vi "Sender UI.vi"(8 "Error In":errorcluster, 9 "Transmission Type":T1, 10 "Transmission Data":string(combo)) -> (0 "Error Out":errorcluster)   [LabVIEW 2023, in "Sender.lvclass"]
uses:
  Sender.lvclass
  Controls/Message Type.ctl
  Controls/Queue Operation.ctl
  Controls/User Event Operations.ctl
  Controls/Messenger Data.ctl
  Controls/Type Class Ref.ctl
  Controls/Class DVR Ref.ctl
  Data/Data.lvclass
  Sender.lvclass/Sender.ctl
  Communication/Communication.lvclass
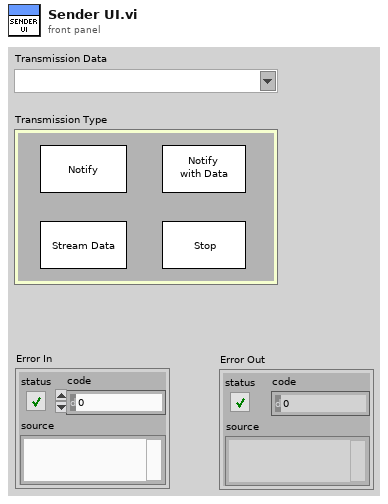
[diagram p1: front panel]
types:
  T1 = typedef "Message Type.ctl" = cluster{"Notify Only":bool, "Notify With Data":bool, "Stream Data":bool, "Hang Up":bool}
  T2 = typedef "Messenger Data.ctl" = cluster{"Message Data path":path, "Start Time":dbl, "Elapsed TIme":dbl, "Message Type":refnum<class "Communication.lvclass">, "Selected Message Data":string, "Selected Message Type":string, "Type DVR Ref":T3[], "Data DVR Ref":T4[], "Type DVR":refnum<data-value>, "Data DVR":refnum<data-value>, "Stream?":bool, "Wait Time":dbl, "Port Number":i32}
  T3 = typedef "Type Class Ref.ctl" = cluster{"Class Name":string, "Class DVR Ref":refnum<data-value>}
  T4 = typedef "Class DVR Ref.ctl" = cluster{"Class DVR Ref":refnum<data-value>, "Class Name":string}
  T5 = typedef "User Event Operations.ctl" = enum16{"Obtain", "Generate", "Destroy"}
  T6 = typedef "Queue Operation.ctl" = enum16{"Create & Enqueue N", "Enqueue N", "Dequeue", "Enstack N", "Flush", "Release"}
  T7 = enum8{"Enabled", "Disabled", "Disabled and Grayed Out"}
  T8 = typedef "Queue Element.ctl" = cluster{"State":string, "Data":variant}
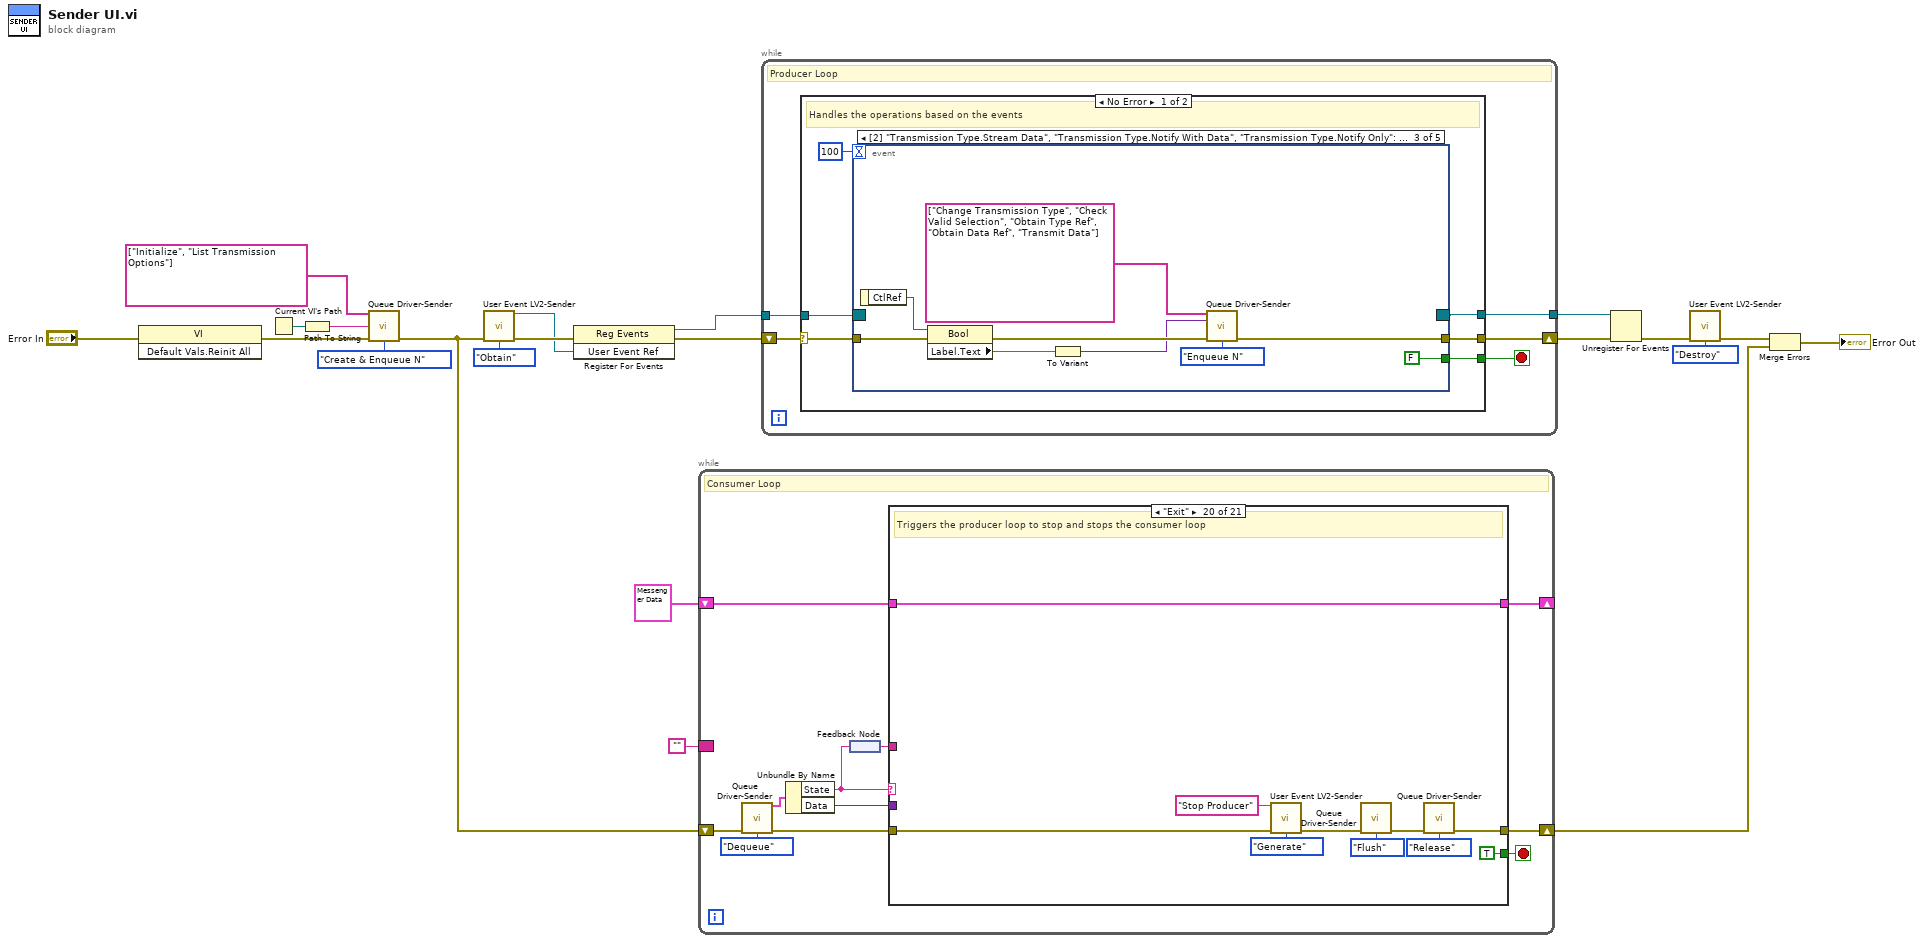
[diagram p0: block diagram]
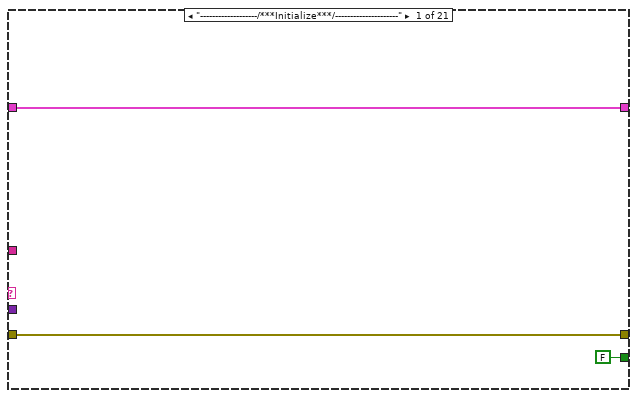
[diagram p2: hidden frame]
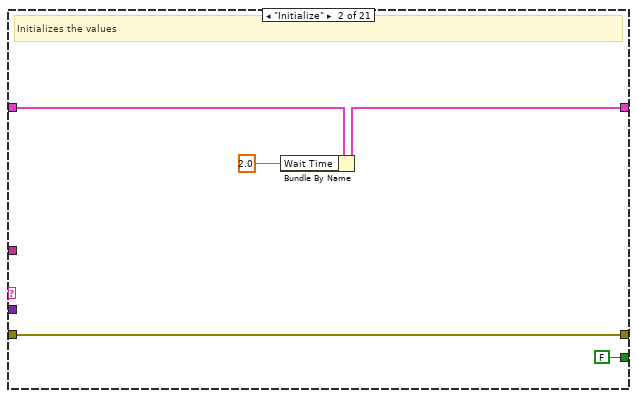
[diagram p3: hidden frame]
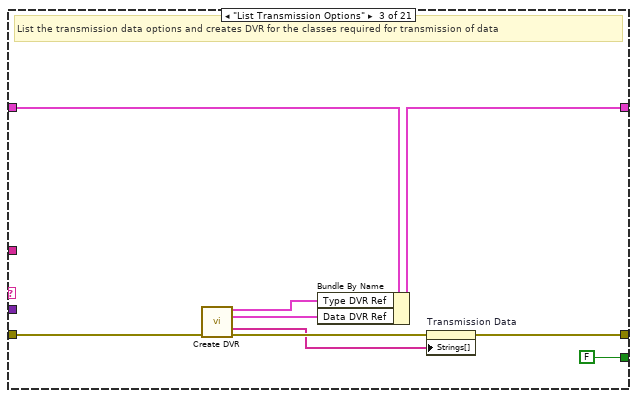
[diagram p4: hidden frame]
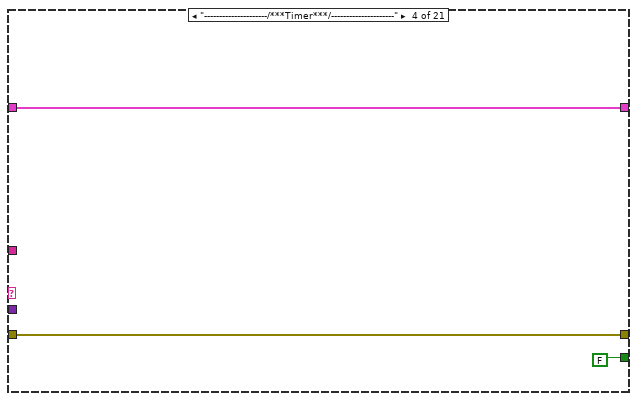
[diagram p5: hidden frame]
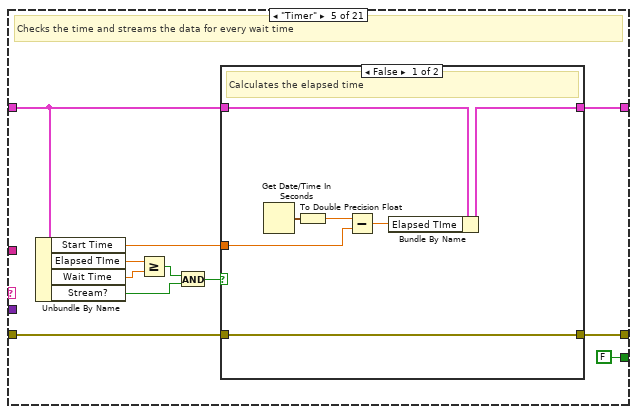
[diagram p6: hidden frame]
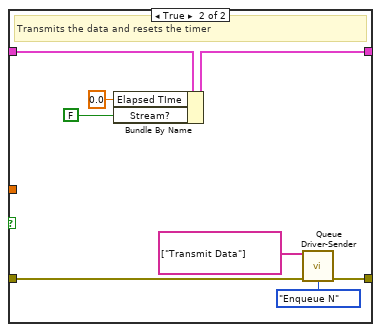
[diagram p7: hidden frame]
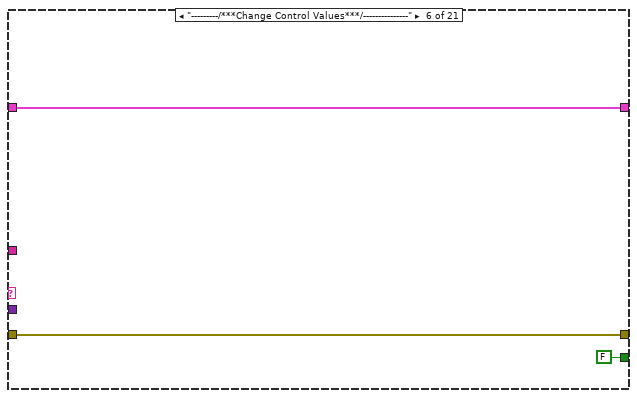
[diagram p8: hidden frame]
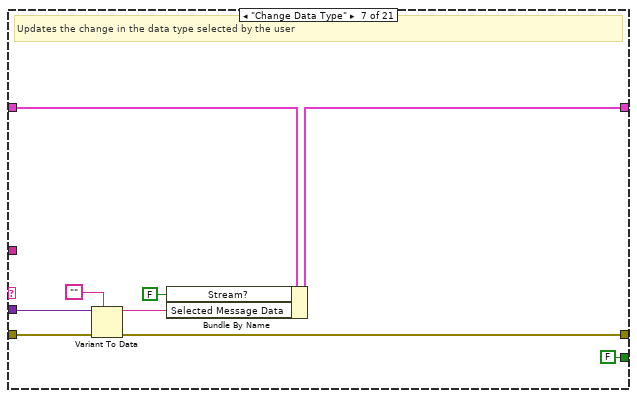
[diagram p9: hidden frame]
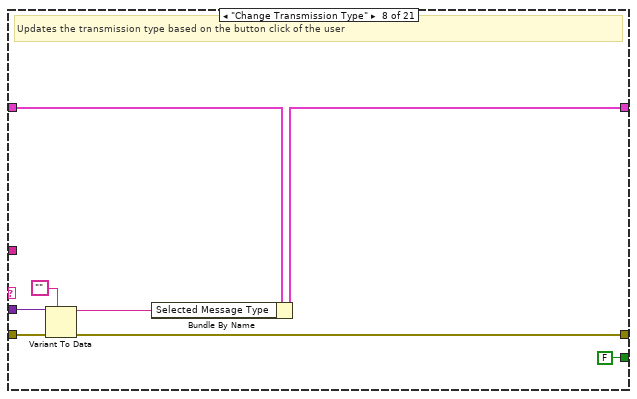
[diagram p10: hidden frame]
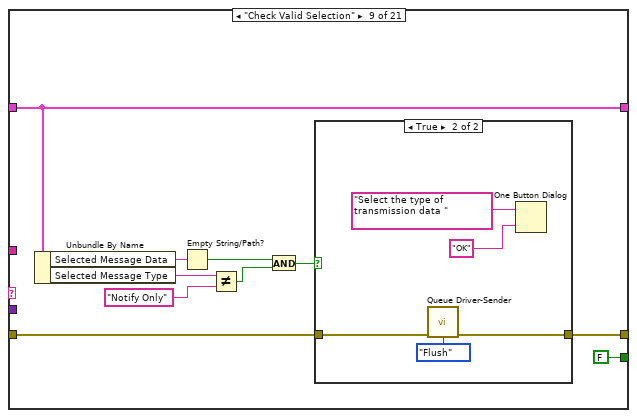
[diagram p11: hidden frame]
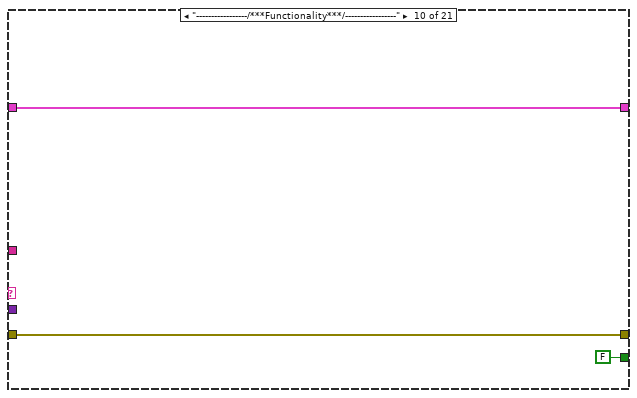
[diagram p13: hidden frame]
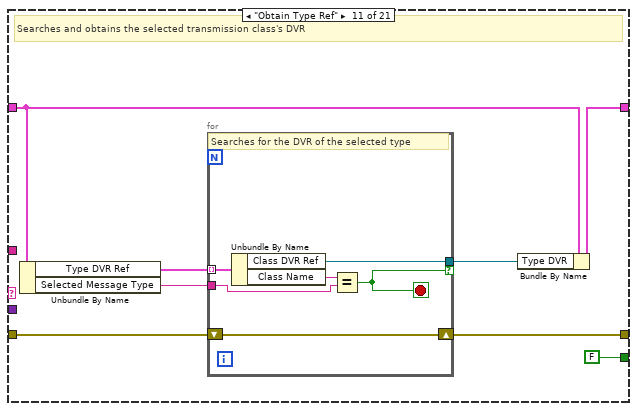
[diagram p14: hidden frame]
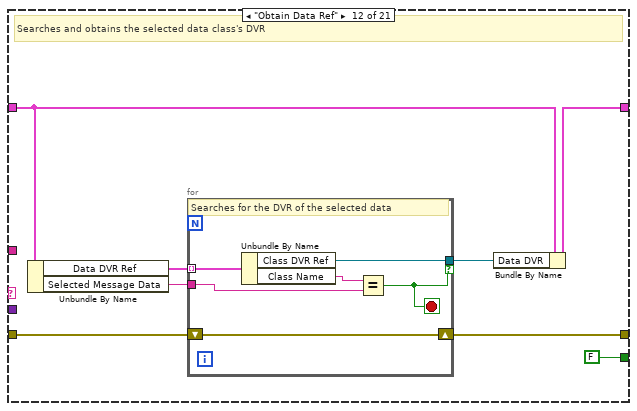
[diagram p15: hidden frame]
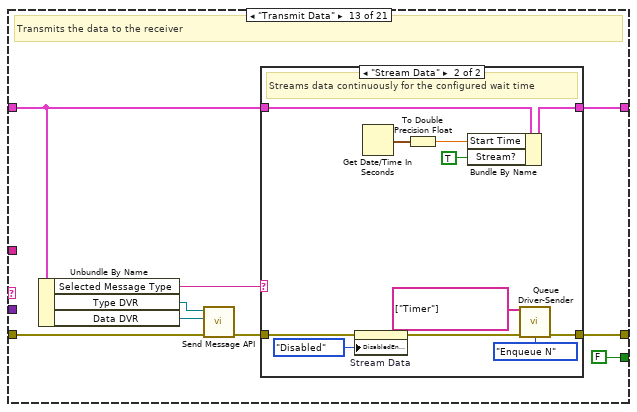
[diagram p16: hidden frame]
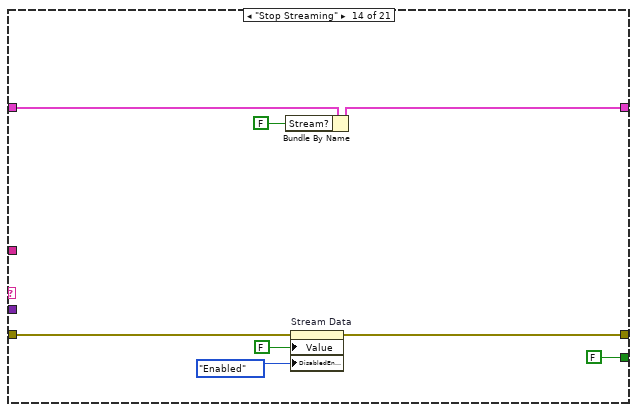
[diagram p18: hidden frame]
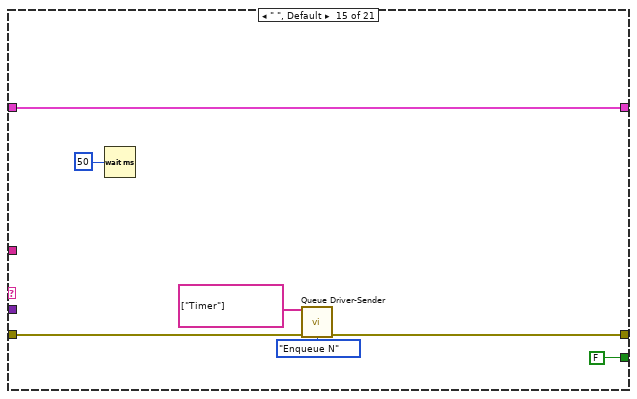
[diagram p19: hidden frame]
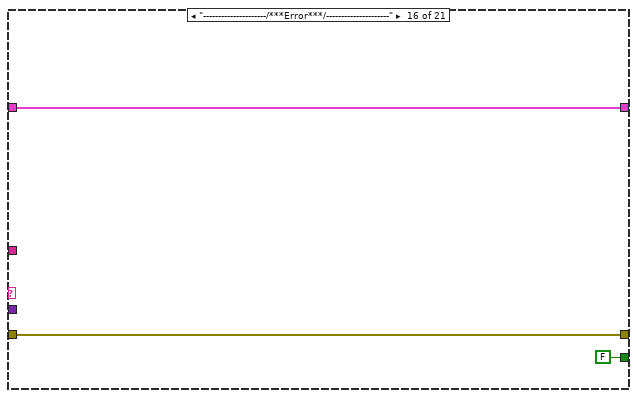
[diagram p20: hidden frame]
diagram:
  n1 = invoke class="VI" method="Default Vals.Reinit All"(error in="Error In") -> (error out=w1:errorcluster)  [unwired: 2 in, 2 out]
  n2 = Current VI's Path() -> (path=w3:path)
  n3 = Path To String(path=w3) -> (string=w2:string)
  n4 = call "Queue Driver-Sender.vi"("States[]"=string[] ["Initialize", "List Transmission Options"], "Queue Name"=w2, "Error In"=w1, "Queue Operation"=Queue_Operation."Create & Enqueue N") -> ("Error Out"=w13:errorcluster)  [unwired: 10 in, 1 out]
  n5 = call "User Event LV2-Sender.vi"("Error In"=w13, "Operation"=User_Event_Operations."Obtain") -> ("User Event Ref"=w11:refnum<user-event>, "Error Out"=w15:errorcluster)  [unwired: 12 in]
  n6 = register-events(error in=w15, w11) -> (reference out=w10:refnum<event-registration>, error out=w12:errorcluster)  [unwired: 1 in]
  n7 = while {
    shift-right: [w31] -> w16
    shift-left: w13 -> [w32]
    border: "" -> [_]
    shift-right: [w22] -> _
    shift-left: T2 {"Message Data path"=path "", "Start Time"=0.0, "Elapsed TIme"=0.0, "Message Type"=refnum, "Selected Message Data"="", "Selected Message Type"="", "Type DVR Ref"=[], "Data DVR Ref"=[], "Type DVR"=refnum, "Data DVR"=refnum, "Stream?"=FALSE, "Wait Time"=0.0, "Port Number"=0} -> [w23]
    stop <- w27 stop-if-true
    # "Consumer Loop"
    n8 = call "Queue Driver-Sender.vi"("Error In"=w32, "Queue Operation"=Queue_Operation."Dequeue") -> ("Dequeue Element"=w28:T8, "Error Out"=w30:errorcluster)  [unwired: 12 in]
    n9 = Unbundle By Name(w28) -> ("State"=w26:string, "Data"=w24:variant)
    n10 = feedback-in #1(w26) -> ()
    n11 = feedback #1() -> (w25:string)
    n12 = case shown="\"Exit\"" w26 {
      tunnel: w30 -> [w35 w39 w49 w52 w63 w81 w90 w98 w108 w117 w125 w139 w154 w175 w182 w185 w191 w220 w228 w238 w247]
      tunnel: [w35 w39 w41 w52 w62 w81 w84 w96 w105 w117 w124 w138 w150 w170 w179 w185 w188 w207 w228 w234 w245] -> w31
      tunnel: [FALSE FALSE FALSE FALSE FALSE FALSE FALSE FALSE FALSE FALSE FALSE FALSE FALSE FALSE FALSE FALSE FALSE FALSE FALSE TRUE FALSE] -> w27
      tunnel: w25 -> [_ _ _ _ _ _ _ _ _ _ _ _ _ _ _ _ w189 _ _ _ _]
      tunnel: w24 -> [_ _ _ _ _ _ w85 w95 _ _ _ _ _ _ _ _ _ w212 _ _ _]
      tunnel: w23 -> [w33 w38 w47 w51 w60 w80 w87 w97 w106 w115 w123 w137 w149 w174 w180 w183 w186 w219 w226 w229 w246]
      tunnel: [w33 w37 w45 w51 w59 w80 w86 w93 w106 w115 w119 w133 w151 w173 w180 w183 w186 w219 w226 w229 w246] -> w22
      frame "-------------------/***Initialize***/---------------------" {
      }
      frame "Initialize" {
        # "Initializes the values"
        n13 = Bundle By Name(cluster=w38, "Wait Time"=2.0) -> (w37:T2)
      }
      frame "List Transmission Options" {
        # "List the transmission data options and creates DVR for the classes required for transmission of data"
        n14 = call "Create DVR.vi"("Error In"=w49) -> ("Communication DVR Refs"=w44:T3[], "Data Type DVR Refs"=w43:T4[], "Data Types"=w42:string[], "Error Out"=w46:errorcluster)  [unwired: 10 in, 1 out]
        n15 = Bundle By Name(cluster=w47, "Type DVR Ref"=w44, "Data DVR Ref"=w43) -> (w45:T2)
        n16 = property on="Transmission Data" class="CmbBox"(error in=w46, "Strings[]"=w42) -> (error out=w41:errorcluster)  [unwired: 1 in, 1 out]
      }
      frame "---------------------/***Timer***/---------------------" {
      }
      frame "Timer" {
        # "Checks the time and streams the data for every wait time"
        n17 = Unbundle By Name(w60) -> ("Start Time"=w61:dbl, "Elapsed TIme"=w57:dbl, "Wait Time"=w53:dbl, "Stream?"=w54:bool)
        n18 = Greater Or Equal?(x=w57, y=w53) -> (x >= y?=w56:bool)
        n19 = And(x=w56, y=w54) -> (x .and. y?=w55:bool)
        n20 = case shown="False" w55 {
          tunnel: w63 -> [w69 w71]
          tunnel: [w69 w77] -> w62
          tunnel: w61 -> [w64 _]
          tunnel: [w68 w74] -> w59
          tunnel: w60 -> [w70 w78]
          frame False {
            # "Calculates the elapsed time"
            n21 = Get Date/Time In Seconds() -> (seconds since 1Jan1904=w67:timestamp)
            n22 = To Double Precision Float(number=w67) -> (double precision float=w65:dbl)
            n23 = Subtract(x=w65, y=w64) -> (x-y=w66:dbl)
            n24 = Bundle By Name(cluster=w70, "Elapsed TIme"=w66) -> (w68:T2)
          }
          frame True {
            # "Transmits the data and resets the timer"
            n25 = Bundle By Name(cluster=w78, "Elapsed TIme"=0.0, "Stream?"=FALSE) -> (w74:T2)
            n26 = call "Queue Driver-Sender.vi"("States[]"=string[] ["Transmit Data"], "Error In"=w71, "Queue Operation"=Queue_Operation."Enqueue N") -> ("Error Out"=w77:errorcluster)  [unwired: 11 in, 1 out]
          }
        }
      }
      frame "---------/***Change Control Values***/---------------" {
      }
      frame "Change Data Type" {
        # "Updates the change in the data type selected by the user"
        n27 = Variant To Data(error in=w90, type="", Variant=w85) -> (data=w83:string, error out=w84:errorcluster)
        n28 = Bundle By Name(cluster=w87, "Stream?"=FALSE, "Selected Message Data"=w83) -> (w86:T2)
      }
      frame "Change Transmission Type" {
        # "Updates the transmission type based on the button click of the user"
        n29 = Variant To Data(error in=w98, type="", Variant=w95) -> (data=w92:string, error out=w96:errorcluster)
        n30 = Bundle By Name(cluster=w97, "Selected Message Type"=w92) -> (w93:T2)
      }
      frame "Check Valid Selection" {
        n31 = Unbundle By Name(w106) -> ("Selected Message Data"=w104:string, "Selected Message Type"=w102:string)
        n32 = Empty String/Path?(string/path=w104) -> (empty?=w101:bool)
        n33 = Not Equal?(x=w102, y="Notify Only") -> (x != y?=w100:bool)
        n34 = And(x=w101, y=w100) -> (x .and. y?=w99:bool)
        n35 = case shown="True" w99 {
          tunnel: w108 -> [w109 w114]
          tunnel: [w109 w111] -> w105
          frame False {
          }
          frame True {
            n36 = call "Queue Driver-Sender.vi"("Error In"=w114, "Queue Operation"=Queue_Operation."Flush") -> ("Error Out"=w111:errorcluster)  [unwired: 12 in, 1 out]
            n37 = One Button Dialog(message="Select the type of transmission data ", button name ("OK")="OK") -> ()  [unwired: 1 out]
          }
        }
      }
      frame "-----------------/***Functionality***/-----------------" {
      }
      frame "Obtain Type Ref" {
        # "Searches and obtains the selected transmission class's DVR"
        n38 = Unbundle By Name(w123) -> ("Type DVR Ref"=w122:T3[], "Selected Message Type"=w121:string)
        n39 = for {
          shift-right: [w131] -> w124
          shift-left: w125 -> [w131]
          tunnel: w122 -> [w130] mode=indexing
          tunnel: w121 -> [w128]
          tunnel: [w127] -> w118 if=w126
          stop <- w126 stop-if-true
          # "Searches for the DVR of the selected type"
          n40 = Unbundle By Name(w130) -> ("Class DVR Ref"=w127:refnum<data-value>, "Class Name"=w129:string)
          n41 = Equal?(x=w129, y=w128) -> (x = y?=w126:bool)
        }
        n42 = Bundle By Name(cluster=w123, "Type DVR"=w118) -> (w119:T2)
      }
      frame "Obtain Data Ref" {
        # "Searches and obtains the selected data class's DVR"
        n43 = Unbundle By Name(w137) -> ("Data DVR Ref"=w136:T4[], "Selected Message Data"=w135:string)
        n44 = for {
          shift-right: [w145] -> w138
          shift-left: w139 -> [w145]
          tunnel: w136 -> [w144] mode=indexing
          tunnel: w135 -> [w141]
          tunnel: [w143] -> w132 if=w140
          stop <- w140 stop-if-true
          # "Searches for the DVR of the selected data"
          n45 = Unbundle By Name(w144) -> ("Class DVR Ref"=w143:refnum<data-value>, "Class Name"=w142:string)
          n46 = Equal?(x=w142, y=w141) -> (x = y?=w140:bool)
        }
        n47 = Bundle By Name(cluster=w137, "Data DVR"=w132) -> (w133:T2)
      }
      frame "Transmit Data" {
        # "Transmits the data to the receiver"
        n48 = Unbundle By Name(w149) -> ("Selected Message Type"=w148:string, "Type DVR"=w147:refnum<data-value>, "Data DVR"=w146:refnum<data-value>)
        n49 = call "Send Message API.vi"("error in (no error)"=w154, "Data DVR"=w146, "Type DVR"=w147) -> ("error out"=w152:errorcluster)  [unwired: 8 in]
        n50 = case shown="\"Stream Data\"" w148 {
          tunnel: w152 -> [w155 w167]
          tunnel: [w156 w166] -> w151
          tunnel: [w155 w163] -> w150
          tunnel: w149 -> [w156 w160]
          frame Default {
          }
          frame "Stream Data" {
            # "Streams data continuously for the configured wait time"
            n51 = property on="Stream Data" class="Bool (strict)"(error in=w167, "DisabledEnum"=T7."Disabled" ("Disabled")) -> (error out=w158:errorcluster)  [unwired: 1 in, 1 out]
            n52 = Get Date/Time In Seconds() -> (seconds since 1Jan1904=w164:timestamp)
            n53 = To Double Precision Float(number=w164) -> (double precision float=w165:dbl)
            n54 = Bundle By Name(cluster=w160, "Start Time"=w165, "Stream?"=TRUE) -> (w166:T2)
            n55 = call "Queue Driver-Sender.vi"("States[]"=string[] ["Timer"], "Error In"=w158, "Queue Operation"=Queue_Operation."Enqueue N") -> ("Error Out"=w163:errorcluster)  [unwired: 11 in, 1 out]
          }
        }
      }
      frame "Stop Streaming" {
        n56 = Bundle By Name(cluster=w174, "Stream?"=FALSE) -> (w173:T2)
        n57 = property on="Stream Data" class="Bool (strict)"(error in=w175, "Value"=FALSE, "DisabledEnum"=T7."Enabled" ("Disabled")) -> (error out=w170:errorcluster)  [unwired: 1 in, 1 out]
      }
      frame " ", Default {
        n58 = Wait (ms)(milliseconds to wait=u32 50) -> ()  [unwired: 1 out]
        n59 = call "Queue Driver-Sender.vi"("States[]"=string[] ["Timer"], "Error In"=w182, "Queue Operation"=Queue_Operation."Enqueue N") -> ("Error Out"=w179:errorcluster)  [unwired: 11 in, 1 out]
      }
      frame "---------------------/***Error***/---------------------" {
      }
      frame "Error" {
        # "Handles the error based on the user acknowledgement"
        n60 = Unbundle By Name(w191) -> ("code"=w193:i32, "source"=w192:string)
        n61 = call <vilib>:"Clear Errors.vi"("error in (no error)"=w191) -> ("error out"=w198:errorcluster)  [unwired: 5 in, 1 out]
        n62 = Format Into String(format string="Error occurred in state \"%s\"!!\nError Code: %d\nError Source: %s\n\nDo you wish to continue?", error in=w198, w189, w193, w192) -> (resulting string=w196:string, error out=w190:errorcluster)  [unwired: 1 in]
        n63 = Two Button Dialog(message=w196, 1:"Exit" ("F button name (\"Cancel\")"), 2:"Continue" ("T button name (\"OK\")")) -> (T button?=w187:bool)
        n64 = case shown="False" w187 {
          tunnel: w190 -> [w203 w204]
          tunnel: [w202 w204] -> w188
          frame False {
            # "Triggers to stop the VI"
            n65 = call "Queue Driver-Sender.vi"("States[]"=string[] ["Exit", "Exit Others"], "Error In"=w203, "Queue Operation"=Queue_Operation."Enstack N") -> ("Error Out"=w202:errorcluster)  [unwired: 11 in, 1 out]
          }
          frame True {
          }
        }
      }
      frame "Producer Error" {
        n66 = Variant To Data(error in=w220, type=errorcluster {"status"=FALSE, "code"=0, "source"=""} ("error out"), Variant=w212) -> (data=w211:errorcluster, error out=w208:errorcluster)
        n67 = Unbundle By Name(w211) -> ("code"=w214:i32, "source"=w213:string)
        n68 = Format Into String(format string="Error occurred in producer loop\nError Code: %d\nError Source: %s\n\nDo you wish to continue?", error in=w208, w214, w213) -> (resulting string=w217:string, error out=w209:errorcluster)  [unwired: 1 in]
        n69 = Two Button Dialog(message=w217, 1:"Exit" ("F button name (\"Cancel\")"), 2:"Continue" ("T button name (\"OK\")")) -> (T button?=w206:bool)
        n70 = case shown="False" w206 {
          tunnel: w209 -> [w223 w225]
          tunnel: [w224 w225] -> w207
          frame False {
            n71 = call "Queue Driver-Sender.vi"("States[]"=string[] ["Exit"], "Error In"=w223, "Queue Operation"=Queue_Operation."Enstack N") -> ("Error Out"=w224:errorcluster)  [unwired: 11 in, 1 out]
          }
          frame True {
          }
        }
      }
      frame "----------------------/***Exit***/----------------------" {
      }
      frame "Exit" {
        # "Triggers the producer loop to stop and stops the consumer loop"
        n72 = call "User Event LV2-Sender.vi"("Event Name"="Stop Producer", "Error In"=w238, "Operation"=User_Event_Operations."Generate") -> ("Error Out"=w232:errorcluster)  [unwired: 11 in, 1 out]
        n73 = call "Queue Driver-Sender.vi"("Error In"=w232, "Queue Operation"=Queue_Operation."Flush") -> ("Error Out"=w236:errorcluster)  [unwired: 12 in, 1 out]
        n74 = call "Queue Driver-Sender.vi"("Error In"=w236, "Queue Operation"=Queue_Operation."Release") -> ("Error Out"=w234:errorcluster)  [unwired: 12 in, 1 out]
      }
      frame "Exit Others" {
        n75 = call "User Event LV2.vi"("Event Name"="", "Error In"=w247, "Operation"=User_Event_Operations."Generate") -> ("Error Out"=w242:errorcluster)  [unwired: 11 in, 1 out]
        n76 = call "User Event LV2-Receive.vi"("Event Name"="Stop", "Error In"=w242, "Operation"=User_Event_Operations."Generate") -> ("Error Out"=w245:errorcluster)  [unwired: 11 in, 1 out]
      }
    }
  }
  n77 = while {
    shift-right: [w250] -> w20
    shift-left: w12 -> [w251]
    tunnel: w10 -> [w249]
    tunnel: [w248] -> w8
    stop <- w252 stop-if-true
    # "Producer Loop"
    n78 = case shown="No Error" w251 {
      selector: w251 -> [w257 w296]
      tunnel: [w258 FALSE] -> w252
      tunnel: [w256 w299] -> w250
      tunnel: w249 -> [w254 _]
      tunnel: [w253 _] -> w248
      frame No Error {
        # "Handles the operations based on the events"
        n79 = event shown="[2] \"Transmission Type.Stream Data\", \"Transmission Type.Notify With Data\", \"Transmission Type.Notify Only\": Value Change" {
          selector: w254 -> [_ _ _ _ _]
          dyn-events: [_ _ _ _ _] -> w253
          timeout: 100 -> [_ _ _ _ _]
          tunnel: [FALSE w262 FALSE FALSE FALSE] -> w258
          tunnel: w257 -> [w259 w264 w282 w287 w294]
          tunnel: [w259 w263 w281 w286 w292] -> w256
          event Timeout {
            # "Waits for any of the events to occur"
            n80 = event-data() -> ()  [unwired: 1 in, 3 out]
          }
          event User Event {
            # "Stops the producer loop"
            n81 = event-data() -> ("State"=w261:string)  [unwired: 1 in]
            n82 = case shown="\"Stop Consumer\"" w261 {
              tunnel: w264 -> [w266 w268 w273]
              tunnel: [w266 w268 w271] -> w263
              tunnel: [FALSE TRUE FALSE] -> w262
              frame Default {
              }
              frame "Stop Producer" {
              }
              frame "Stop Consumer" {
                # "Initiates to stop the consumer loop"
                n83 = call "Queue Driver-Sender.vi"("States[]"=string[] ["Exit"], "Error In"=w273, "Queue Operation"=Queue_Operation."Enstack N") -> ("Error Out"=w271:errorcluster)  [unwired: 11 in, 1 out]
              }
            }
          }
          event Value Change {
            n84 = event-data() -> ("CtlRef"=w277:refnum<vi>)  [unwired: 1 in]
            n85 = property class="Bool"(reference=w277, error in=w282) -> (error out=w278:errorcluster, "Label.Text"=w275:string)  [unwired: 1 out]
            n86 = To Variant(anything=w275) -> (Variant=w274:variant)
            n87 = call "Queue Driver-Sender.vi"("States[]"=string[] ["Change Transmission Type", "Check Valid Selection", "Obtain Type Ref", "Obtain Data Ref", "Transmit Data"], "Data"=w274, "Error In"=w278, "Queue Operation"=Queue_Operation."Enqueue N") -> ("Error Out"=w281:errorcluster)  [unwired: 10 in, 1 out]
          }
          event Value Change {
            n88 = event-data() -> ()  [unwired: 1 in, 1 out]
            n89 = call "Queue Driver-Sender.vi"("States[]"=string[] ["Stop Streaming"], "Error In"=w287, "Queue Operation"=Queue_Operation."Enqueue N") -> ("Error Out"=w286:errorcluster)  [unwired: 11 in, 1 out]
          }
          event "Transmission Data": Value Change {
            n90 = event-data() -> ("NewVal"=w291:string)  [unwired: 1 in]
            n91 = To Variant(anything=w291) -> (Variant=w289:variant)
            n92 = call "Queue Driver-Sender.vi"("States[]"=string[] ["Change Data Type"], "Data"=w289, "Error In"=w294, "Queue Operation"=Queue_Operation."Enqueue N") -> ("Error Out"=w292:errorcluster)  [unwired: 10 in, 1 out]
          }
        }
      }
      frame Error {
        # "Captures the error and sends to the consumer loop to handle"
        n93 = call <vilib>:"Clear Errors.vi"("error in (no error)"=w296) -> ("error out"=w300:errorcluster)  [unwired: 5 in, 1 out]
        n94 = To Variant(anything=w296) -> (Variant=w295:variant)
        n95 = call "Queue Driver-Sender.vi"("States[]"=string[] ["Exit Producer"], "Data"=w295, "Error In"=w300, "Queue Operation"=Queue_Operation."Enstack N") -> ("Error Out"=w299:errorcluster)  [unwired: 10 in, 1 out]
      }
    }
  }
  n96 = Unregister For Events(event registration refnum=w8, error in=w20) -> (error out=w9:errorcluster)
  n97 = call "User Event LV2-Sender.vi"("Error In"=w9, "Operation"=User_Event_Operations."Destroy") -> ("Error Out"=w7:errorcluster)  [unwired: 12 in, 1 out]
  n98 = Merge Errors(w7, w16) -> (→"Error Out":errorcluster)
